vi "Initialize Label Buffers.vi"(8 "error in":errorcluster, 10 "module handle":u8, 11 "Rx channels in":T1[](array[typedef]) {"labels settings for RT"."Label Timestamp Channel Data Reference" format="%.0x"; "labels settings for RT"."Word Initial Raw Value" format="%032.0f"; "labels settings for RT"."Label Disable/Trigger Channel Reference" format="%.0x"; "labels settings for RT"."parameter driver data"."Tx parameter refs" format="%.0x"; "labels settings for RT"."SDI" format="%02b"; "labels settings for RT"."label" format="%.0o"}) -> (0 "error out":errorcluster, 3 "Rx channels out":T1[](array[typedef]) {"labels settings for RT"."Label Timestamp Channel Data Reference" format="%.0x"; "labels settings for RT"."Word Initial Raw Value" format="%032.0f"; "labels settings for RT"."Label Disable/Trigger Channel Reference" format="%.0x"; "labels settings for RT"."parameter driver data"."Tx parameter refs" format="%.0x"; "labels settings for RT"."SDI" format="%02b"; "labels settings for RT"."label" format="%.0o"})   [LabVIEW 2024, in "AIM ARINC 429 Hardware API.lvlib"]
uses:
  AIM ARINC 429 Hardware API.lvlib
  Shared/RT Hardware Channel Settings.ctl
  Shared/RT Label Settings.ctl
  Shared/Label.ctl
  Shared/RT Parameters.ctl
  Shared/Parameter Definition.ctl
  <vilib>/NI/NI VeriStand Encoding and Decoding/Encoding.ctl
  <vilib>/NI VeriStand/Custom Device API/Custom Device Item Ref.ctl
  Shared/Transfer Type.ctl
  <vilib>/NI VeriStand/Custom Device API/Data Reference.ctl
  Shared/Transfer Speed.ctl
  <instrlib>/AIM GmbH/_ARINC-429/subvi/Error Converter (ErrCode or Status).vi
  <instrlib>/AIM GmbH/_ARINC-429/subvi/Get Library Path.vi
  <instrlib>/AIM GmbH/_ARINC-429/VIs/Library/Api429Lib Error Desc Get.vi
  <instrlib>/AIM GmbH/_ARINC-429/subvi/Get Error Number Offset.vi
  <vilib>/Utility/error.llb/Error Cluster From Error Code.vi
  <instrlib>/AIM GmbH/_ARINC-429/AIM429LV.lvlib
  <vilib>/NI/NI VeriStand Encoding and Decoding/Encoding and Decoding.lvlib
  <vilib>/NI VeriStand/Custom Device API/Custom Device API.lvlib
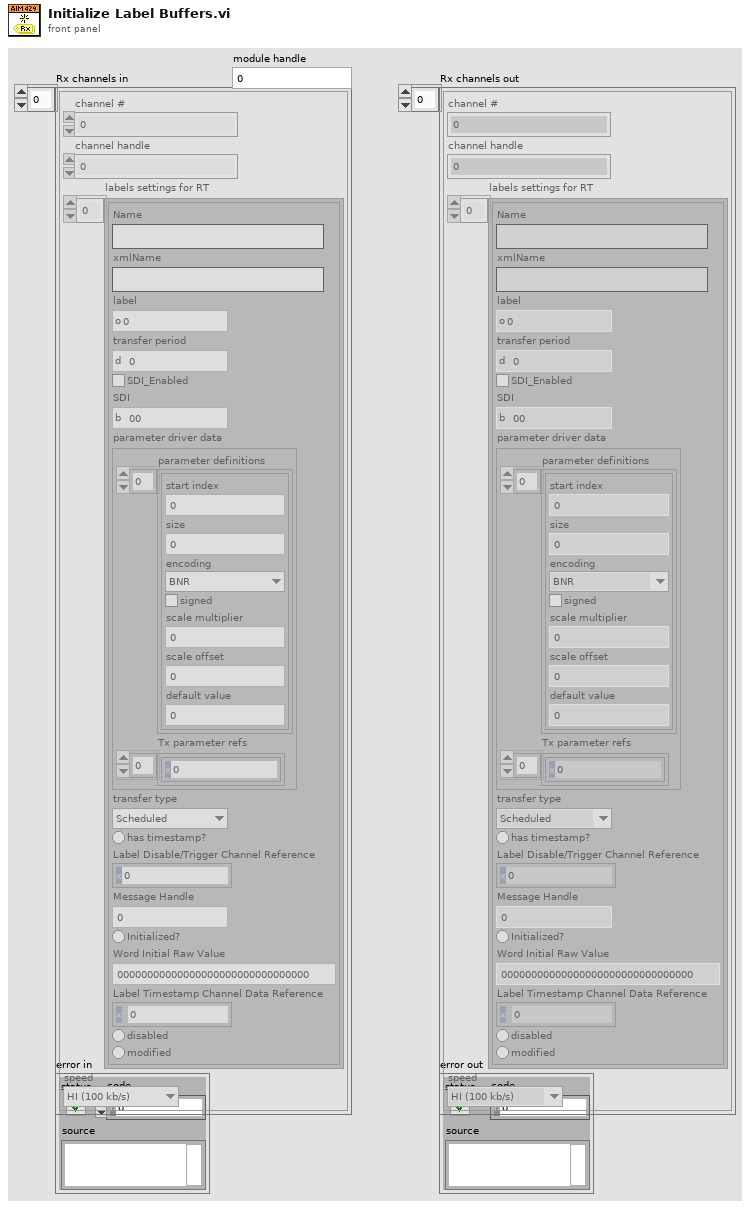
[diagram p1: front panel]
types:
  T1 = typedef "RT Hardware Channel Settings.ctl" = cluster{"channel #":u16, "channel handle":u64, "labels settings for RT":T2[], "speed":T10}
  T2 = typedef "RT Label Settings.ctl" = cluster{"Name":string, "xmlName":string, "label":T3, "transfer period":u32, "SDI_Enabled":bool, "SDI":u8, "parameter driver data":T4, "transfer type":T8, "has timestamp?":bool, "Label Disable/Trigger Channel Reference":T7, "Message Handle":u64, "Initialized?":bool, "Word Initial Raw Value":u32, "Label Timestamp Channel Data Reference":T9, "disabled":bool, "modified":bool}
  T3 = typedef "Label.ctl" = u8
  T4 = typedef "RT Parameters.ctl" = cluster{"parameter definitions":T5[], "Tx parameter refs":T7[]}
  T5 = typedef "Parameter Definition.ctl" = cluster{"start index":i32, "size":i32, "encoding":T6, "signed":bool, "scale multiplier":dbl, "scale offset":dbl, "default value":dbl}
  T6 = typedef "Encoding and Decoding.lvlib/Encoding.ctl" = enum16{"BNR", "BCD", "Discrete"}
  T7 = typedef "Custom Device API.lvlib/Custom Device Item Ref.ctl" = u64
  T8 = typedef "Transfer Type.ctl" = enum16{"Scheduled", "Acyclic", "Block", "Strobe"}
  T9 = typedef "Custom Device API.lvlib/Data Reference.ctl" = i32
  T10 = typedef "Transfer Speed.ctl" = enum16{"LO (12.5 kb/s)", "HI (100 kb/s)"}
  T11 = cluster{"label":u32, "sdi":u32, "con":u32, "irCon":u32, "irIndex":u32, "bufSize":u32}
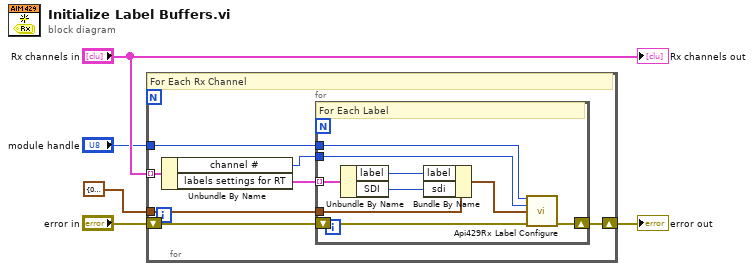
[diagram p0: block diagram]
diagram:
  n1 = for {
    tunnel: "Rx channels in" -> [w12] mode=indexing
    shift-right: [w9] -> w3
    shift-left: "error in" -> [w11]
    tunnel: "module handle" -> [w8]
    tunnel: T11 {"label"=0, "sdi"=0, "con"=0, "irCon"=0, "irIndex"=0, "bufSize"=0} ("label_setup") -> [w6]
    # "For Each Rx Channel"
    n2 = Unbundle By Name(w12) -> ("channel #"=w7:u16, "labels settings for RT"=w10:T2[])
    n3 = for {
      shift-right: [w15] -> w9
      shift-left: w11 -> [w20]
      tunnel: w8 -> [w21]
      tunnel: w7 -> [w19]
      tunnel: w10 -> [w18] mode=indexing
      tunnel: w6 -> [w14]
      # "For Each Label"
      n4 = Unbundle By Name(w18) -> ("label"=w17:T3, "SDI"=w16:u8)
      n5 = Bundle By Name(cluster=w14, "label"=w17, "sdi"=w16) -> (w13:T11)
      n6 = call <instrlib>:"Api429Rx Label Configure.vi"("board_handle"=w21, "b_Chn"=w19, "label_setup"=w13, "error in (no error)"=w20) -> ("error out"=w15:errorcluster)  [unwired: 9 in, 2 out]
    }
  }
  "error out" <- w3
  "Rx channels out" <- "Rx channels in"
